vi "Set Wheel Separations.vi"(8 "error in (no error)":errorcluster, 9 "wheel separation length":dbl=1.5, 10 "wheel separation width":dbl=1.0, 11 "ackermann steering frame in":refnum<class "NI_Robotics_Ackermann Steering Frame.lvclass">) -> (0 "error out":errorcluster, 3 "ackermann steering frame out":refnum<class "NI_Robotics_Ackermann Steering Frame.lvclass">)   [LabVIEW 2017, in "NI_Robotics_Ackermann Steering Frame.lvclass"]
uses:
  <vilib>/robotics/Steering/Ackermann Steering Frame/NI_Robotics_Ackermann Steering Frame.lvclass
  c:/Program Files (x86)/National Instruments/LabVIEW 2017/vi.lib/robotics/Steering/Steering Frame/NI_Robotics_Steering Frame.lvclass
  <vilib>/robotics/Steering/Steering Frame/NI_Robotics_Steering Frame.lvclass/NI_Robotics_Steering Frame.ctl
  <vilib>/robotics/Steering/Wheel/NI_Robotics_Wheel.lvclass/NI_Robotics_Wheel.ctl
  <vilib>/robotics/Steering/Ackermann Steering Frame/NI_Robotics_Ackermann Steering Frame.lvclass/NI_Robotics_Ackermann Steering Frame.ctl
  <vilib>/robotics/Steering/Wheel/Update Steering to Wheel Frame Transform.vi
  <vilib>/Analysis/coordinate.llb/Wrap Angle.vi
  <vilib>/Analysis/coordinate.llb/Wrap Angle (scalar).vi
  <vilib>/robotics/Steering/Steering Frame/NI_Robotics_Steering Frame.lvclass
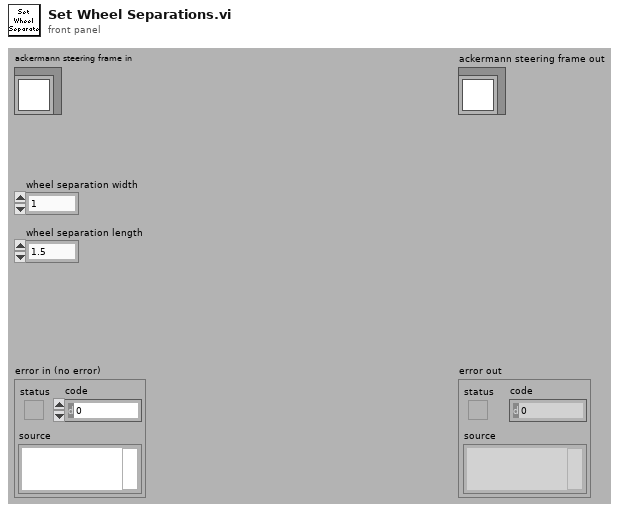
[diagram p1: front panel]
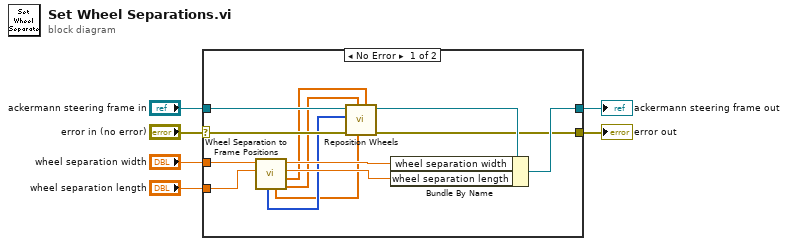
[diagram p0: block diagram]
diagram:
  n1 = case shown="No Error" "error in (no error)" {
    selector: "error in (no error)" -> [w18 w21]
    tunnel: [w13 w21] -> w5
    tunnel: [w14 w20] -> w3
    tunnel: "ackermann steering frame in" -> [w19 w20]
    tunnel: "wheel separation width" -> [w17 _]
    tunnel: "wheel separation length" -> [w16 _]
    frame No Error {
      n2 = call <vilib>:"Wheel Separation to Frame Positions.vi"("wheel separation length"=w16, "wheel separation width"=w17) -> ("wheel y positions"=w9:dbl[], "wheel x positions"=w10:dbl[], "coerced wheel separation length"=w11:dbl, "coerced wheel separation width"=w12:dbl, "wheel frame angles (rad)"=w7:dbl[], "wheel indexes"=w8:i32[])  [unwired: 4 in]
      n3 = call <vilib>:"Reposition Wheels.vi"("x positions"=w10, "frame angles (rad)"=w7, "y positions"=w9, "error in (no error)"=w18, "wheel indexes"=w8, "steering frame in"=w19) -> ("error out"=w13:errorcluster, "steering frame out"=w15:refnum<class "NI_Robotics_Ackermann Steering Frame.lvclass">)  [unwired: 3 in, 1 out]
      n4 = Bundle By Name(cluster=w15, "wheel separation width"=w12, "wheel separation length"=w11) -> (w14:refnum<class "NI_Robotics_Ackermann Steering Frame.lvclass">)
    }
    frame Error {
    }
  }
  "error out" <- w5
  "ackermann steering frame out" <- w3
